vi "Execute.vi"(0 "reference in":refnum<class "Spindle.lvclass">, 5 "error in (no error)":errorcluster) -> (14 "reference out":refnum<class "Spindle.lvclass">, 19 "error out":errorcluster)   [LabVIEW 2013, in "Spindle.lvclass"]
uses:
  Spindle.lvclass
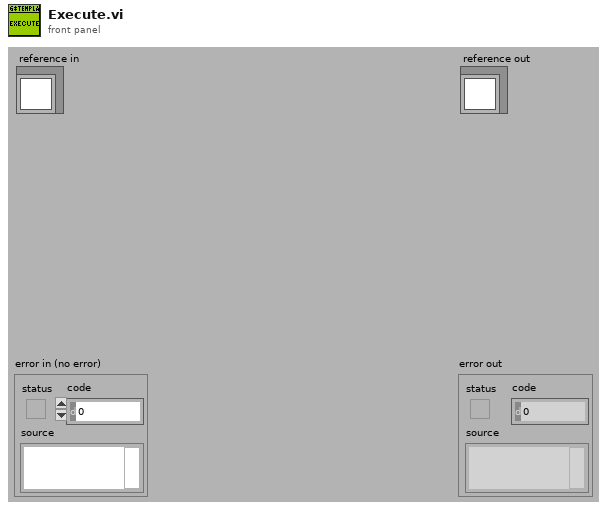
[diagram p1: front panel]
types:
  T1 = typedef "Spindle.lvclass/ObjectAttributes.ctl" = cluster{"MyAttribute":dbl}
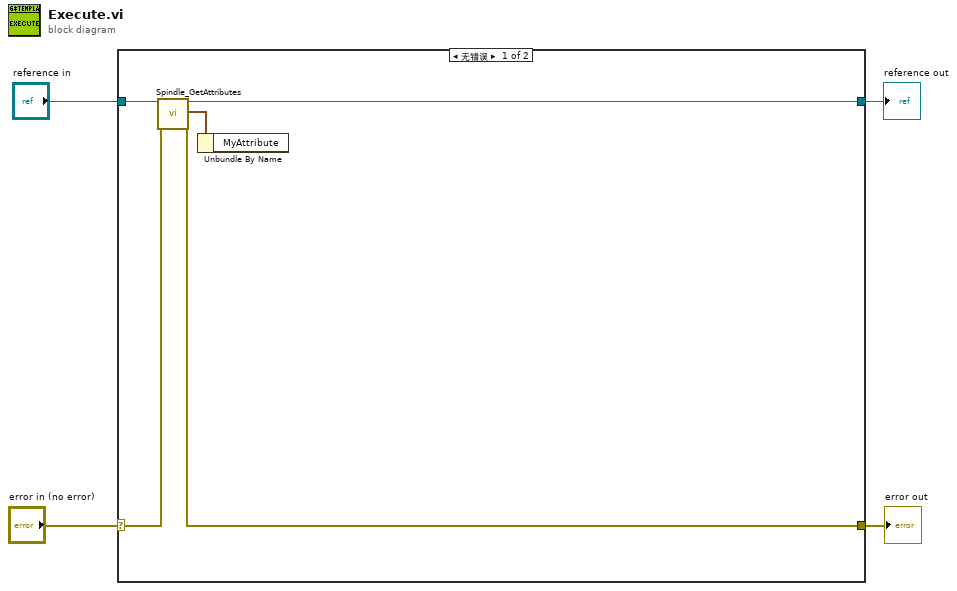
[diagram p0: block diagram]
diagram:
  n1 = case shown="无错误" "error in (no error)" {
    selector: "error in (no error)" -> [w9 w11]
    tunnel: [w8 w11] -> w3
    tunnel: [w7 w10] -> w1
    tunnel: "reference in" -> [w5 w10]
    frame No Error {
      n2 = call "Spindle_GetAttributes.vi"("reference in"=w5, "error in (no error)"=w9) -> ("reference out"=w7:refnum<class "Spindle.lvclass">, "attributes"=w6:T1, "error out"=w8:errorcluster)  [unwired: 14 in, 1 out]
      n3 = Unbundle By Name(w6) -> ()  [unwired: 1 out]
    }
    frame Error {
    }
  }
  "error out" <- w3
  "reference out" <- w1
